vi "Pump waveplate.vi"(0 "VISA Refnum in":refnum<visa-resource-name>, 1 "Trigger rate \nat maximum":dbl, 2 "Mode":enum16{"Constant power", "Constant time"}(ring), 3 "Trigger rate warnings?":bool, 5 "Target trial \nlength (ms)":dbl, 7 "Target trigger rate":dbl, 8 "Threshold":dbl, 9 "Photon #":i32, 11 "error in (no error)":errorcluster, 12 "appended array":dbl[][](array[numeric]), 13 "N":i32=5, 14 "Axis in":i32=3) -> (4 "VISA Refnum out":refnum<visa-resource-name>, 6 "Current position (units)":dbl, 10 "WP Error":bool=TRUE, 15 "error out":errorcluster)   [LabVIEW 2013]
uses:
  <vilib>/imath/engines/lvmath2/RunTimeEngine/NodeEndStatement/NIMS_NodeEndStatement_Output.vi
  <instcachedir>/0/NIMS_NodeEndStatement_Output_53EC0D466D134D7ABD903AC30B43404B.lvgen/NIMS_NodeEndStatement_Output_53EC0D466D134D7ABD903AC30B43404B_010.vi
  <instcachedir>/0/NIMS_NodeEndStatement_Output_53EC0D466D134D7ABD903AC30B43404B.lvgen/NIMS_NodeEndStatement_Output_53EC0D466D134D7ABD903AC30B43404B_009.vi
  <vilib>/imath/engines/lvmath2/RunTimeEngine/BuiltInFunctions/asin/NIMS_asin(C).vi
  <instcachedir>/0/NIMS_asin(C)_73B68F6B04904A8785972686F67E90FD.lvgen/NIMS_asin(C)_73B68F6B04904A8785972686F67E90FD_001.vi
  <vilib>/imath/engines/lvmath2/RunTimeEngine/BuiltInFunctions/abs/NIMS_abs(signed).vi
  <instcachedir>/0/NIMS_abs(signed)_C4FCB8E6058B49B797C7C8D53CA5F6EC.lvgen/NIMS_abs(signed)_C4FCB8E6058B49B797C7C8D53CA5F6EC_002.vi
  <vilib>/imath/engines/lvmath2/RunTimeEngine/ErrorHandling/NIMS_Finalize Error.vi
  <instcachedir>/0/NIMS_NodeEndStatement_Output_53EC0D466D134D7ABD903AC30B43404B.lvgen/NIMS_NodeEndStatement_Output_53EC0D466D134D7ABD903AC30B43404B_001.vi
  <instcachedir>/0/NIMS_abs(signed)_C4FCB8E6058B49B797C7C8D53CA5F6EC.lvgen/NIMS_abs(signed)_C4FCB8E6058B49B797C7C8D53CA5F6EC_000.vi
panel:
  in  "Number of trials to skip":i32=10
  out "Calculated trial length":dbl
  out "angle":dbl
  out "theta1":dbl
  out "t_ratio":dbl
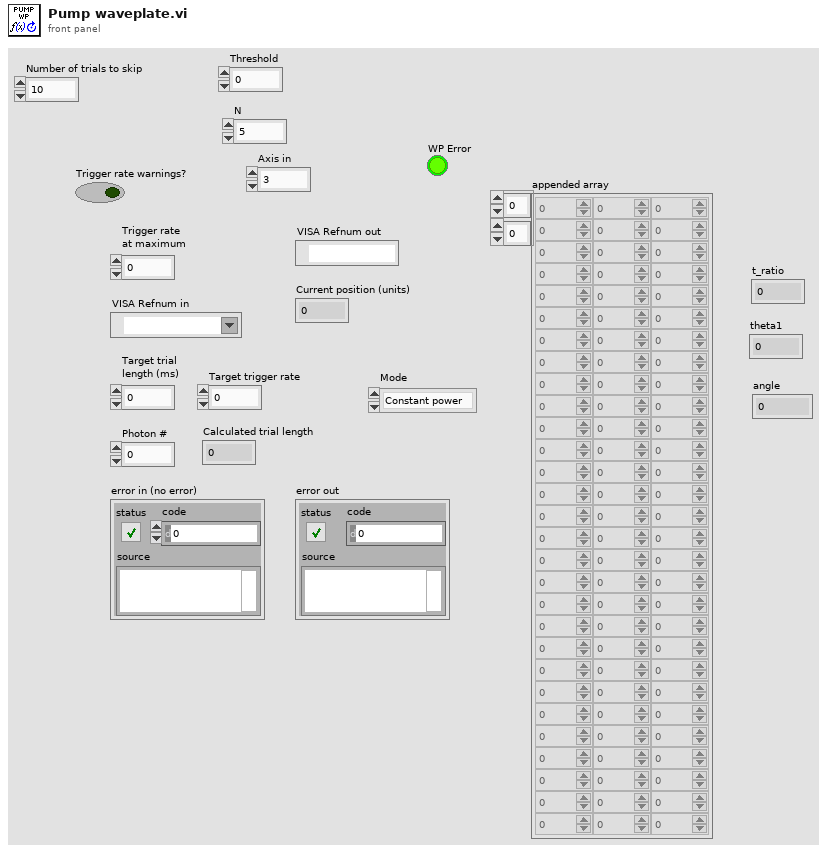
[diagram p1: front panel]
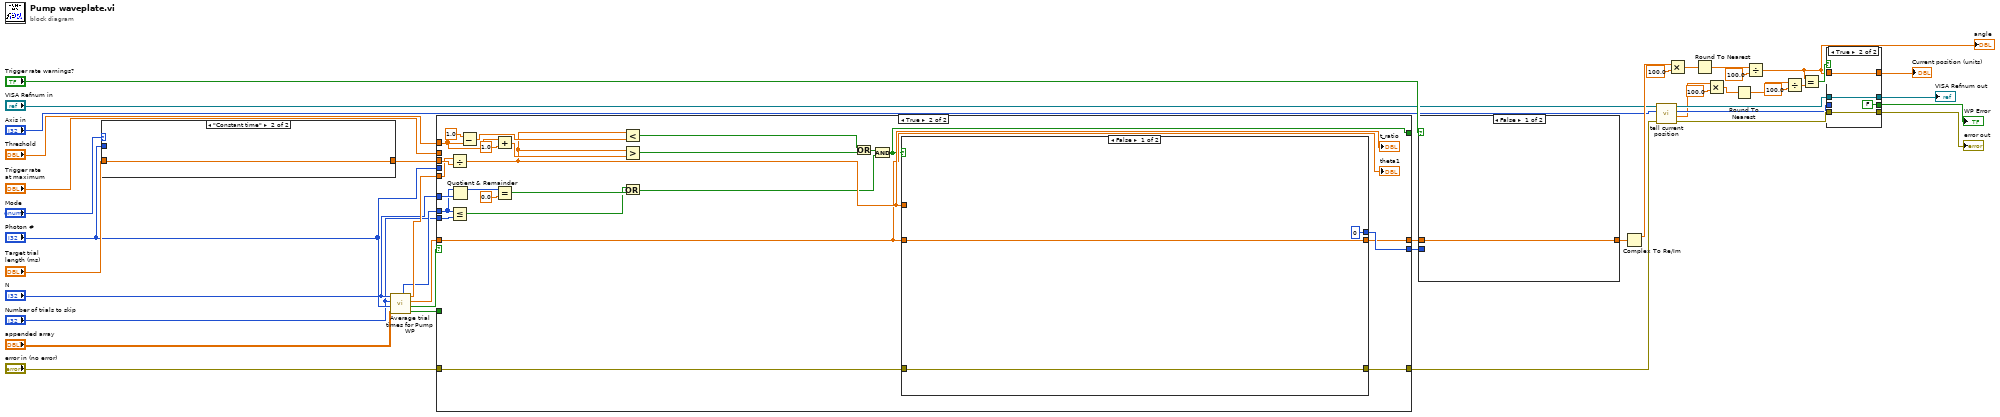
[diagram p0: block diagram]
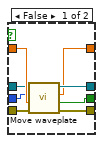
[diagram p2: hidden frame]
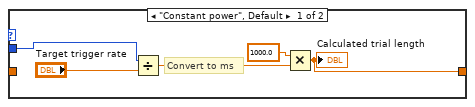
[diagram p3: hidden frame]
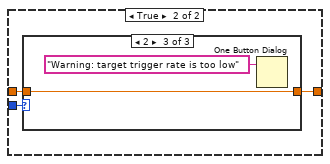
[diagram p4: hidden frame]
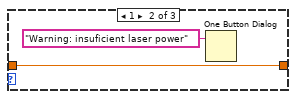
[diagram p6: hidden frame]
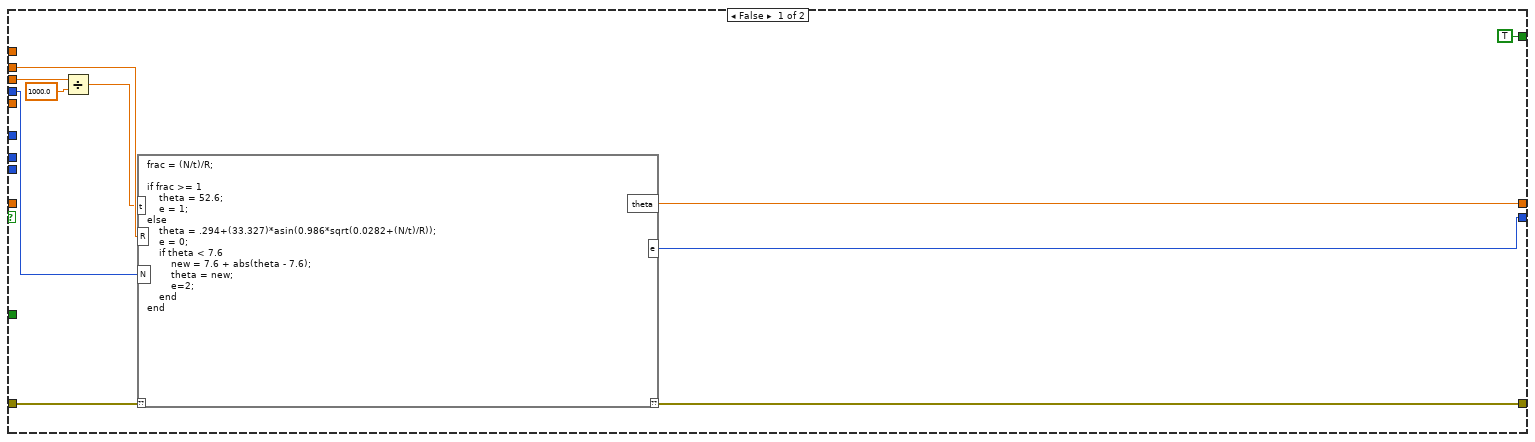
[diagram p7: hidden frame]
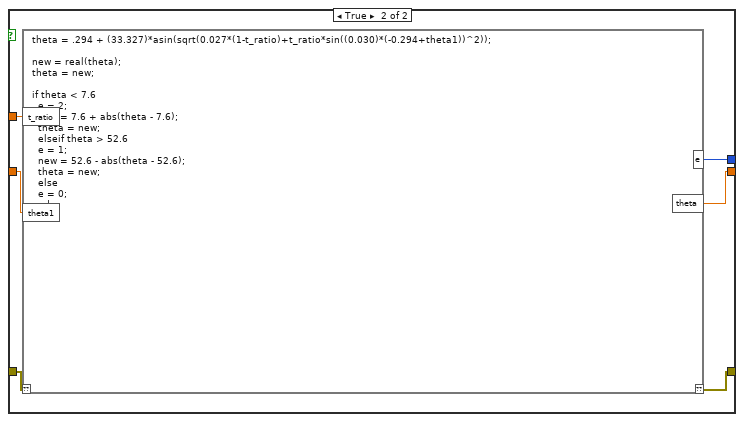
[diagram p8: hidden frame]
diagram:
  n1 = case shown="\"Constant time\"" "Mode" {
    tunnel: [w43 w48] -> w27
    tunnel: "Target trial \nlength (ms)" -> [_ w48]
    tunnel: "Photon #" -> [w47 _]
    frame "Constant power", Default {
      # "Convert to ms"
      n2 = Divide(x=w47, y="Target trigger rate") -> (x/y=w45:dbl)
      n3 = Multiply(x=1000.0, y=w45) -> (x*y=w43:dbl)
      "Calculated trial length" <- w43
    }
    frame "Constant time" {
    }
  }
  n4 = call "Average trial times for Pump WP.vi"("appended array"="appended array", "Photon #"="Photon #", "Number of trials to skip"="Number of trials to skip", "N"="N") -> ("At least N+1 values?"=w21:bool, "At least 1 value?"=w20:bool, "Last WP angle"=w19:dbl, "Output"=w18:dbl, "Number of values with specified photon #"=w17:i16)  [unwired: 1 in]
  n5 = case shown="True" w20 {
    tunnel: "Trigger rate \nat maximum" -> [w58 _]
    tunnel: [w50 w195] -> w39
    tunnel: [w57 w198] -> w41
    tunnel: w27 -> [w52 w199]
    tunnel: "Photon #" -> [w56 _]
    tunnel: "error in (no error)" -> [w55 w197]
    tunnel: [w54 w196] -> w14
    tunnel: "Threshold" -> [_ w191]
    tunnel: w21 -> [_ _]
    tunnel: w19 -> [_ w185]
    tunnel: w18 -> [_ w189]
    tunnel: [TRUE w184] -> _
    tunnel: w17 -> [_ w177]
    tunnel: "N" -> [_ w180]
    tunnel: "Number of trials to skip" -> [_ w176]
    frame False {
      n6 = Divide(x=w52, y=1000.0) -> (x/y=w51:dbl)
      n7 = mathscript code="frac = (N/t)/R;\n\nif frac >= 1\n    theta = 52.6;\n    e = 1;\nelse\n    theta = .294+(33.327)*asin(0.986*sqrt(0.0282+(N/t)/R));\n    e = 0;\n    if theta < 7.6\n        new = 7.6 + abs(theta - 7.6);\n        theta = new;\n        e=2;\n    end\nend"("??"=w55, "t"=w51, "R"=w58, "N"=w56) -> ("??"=w54:errorcluster, "e"=w57:i32, "theta"=w50:cdb)
    }
    frame True {
      n8 = Divide(x=w189, y=w199) -> (x/y=w188:dbl)
      "t_ratio" <- w188
      n9 = Less Or Equal?(x=w177, y=w176) -> (x <= y?=w175:bool)
      n10 = Quotient & Remainder(x=w177, y=w180) -> (x-y*floor(x/y)=w182:i32)  [unwired: 1 out]
      n11 = Subtract(x=1.0 ("y"), y=w191) -> (x-y=w190:dbl)
      n12 = Add(x=w191, y=1.0) -> (x+y=w193:dbl)
      n13 = Equal?(x=w182, y=0.0) -> (x = y?=w179:bool)
      n14 = Less?(x=w188, y=w190) -> (x < y?=w186:bool)
      n15 = Greater?(x=w188, y=w193) -> (0:w187:bool)
      n16 = Or(x=w175, y=w179) -> (x .or. y?=w178:bool)
      n17 = Or(x=w186, y=w187) -> (x .or. y?=w183:bool)
      n18 = And(x=w183, y=w178) -> (x .and. y?=w184:bool)
      n19 = case shown="False" w184 {
        tunnel: w188 -> [_ w208]
        tunnel: [0 ("e") w207] -> w198
        tunnel: w197 -> [w201 w206]
        tunnel: [w201 w205] -> w196
        tunnel: [w200 w204] -> w195
        tunnel: w185 -> [w200 w203]
        frame False {
        }
        frame True {
          n20 = mathscript code="theta = .294 + (33.327)*asin(sqrt(0.027*(1-t_ratio)+t_ratio*sin((0.030)*(-0.294+theta1))^2));\n\nnew = real(theta);\ntheta = new;\n\nif theta < 7.6\n  e = 2;\n  new = 7.6 + abs(theta - 7.6);\n  theta = new;\n  elseif theta > 52.6\n  e = 1;\n  new = 52.6 - abs(theta - 52.6);\n  theta = new;\n  else\n  e = 0;\nend"("??"=w206, "t_ratio"=w208, "theta1"=w203) -> ("??"=w205:errorcluster, "e"=w207:i32, "theta"=w204:dbl)
        }
      }
      "theta1" <- w185
    }
  }
  n21 = case shown="False" "Trigger rate warnings?" {
    tunnel: [w336 w339] -> w38
    tunnel: w39 -> [w336 w338]
    tunnel: w41 -> [_ w337]
    frame False {
    }
    frame True {
      n22 = case shown="2" w337 {
        tunnel: w338 -> [w340 w341 w343]
        tunnel: [w340 w341 w343] -> w339
        frame 0, Default {
        }
        frame 1 {
          n23 = One Button Dialog(message="Warning: insuficient laser power") -> ()  [unwired: 1 in, 1 out]
        }
        frame 2 {
          n24 = One Button Dialog(message="Warning: target trigger rate is too low") -> ()  [unwired: 1 in, 1 out]
        }
      }
    }
  }
  n25 = Complex To Re/Im(x + iy=w38) -> (x=w37:dbl)  [unwired: 1 out]
  n26 = call "tell current position.vi"("error in"=w14, "Axis in"="Axis in", "VISA Handle in"="VISA Refnum in") -> ("error out"=w13:errorcluster, "Current position (units)"=w2:dbl, "Axis out"=w10:i32, "VISA Handle out"=w9:refnum<visa-resource-name>)  [unwired: 2 in, 1 out]
  n27 = Multiply(x=w37, y=100.0) -> (x*y=w35:dbl)
  n28 = Round To Nearest(number=w35) -> (nearest integer value=w34:dbl)
  n29 = Multiply(x=w2, y=100.0) -> (x*y=w5:dbl)
  n30 = Round To Nearest(number=w5) -> (nearest integer value=w4:dbl)
  n31 = Divide(x=w34, y=100.0) -> (x/y=w7:dbl)
  "angle" <- w7
  n32 = Divide(x=w4, y=100.0) -> (x/y=w1:dbl)
  n33 = Equal?(x=w7, y=w1) -> (x = y?=w8:bool)
  n34 = case shown="True" w8 {
    tunnel: w13 -> [w352 w356]
    tunnel: w7 -> [w351 w353]
    tunnel: w10 -> [w350 _]
    tunnel: w9 -> [w349 w354]
    tunnel: [w348 w354] -> w31
    tunnel: [w347 FALSE ("WP Error")] -> w30
    tunnel: [w346 w353] -> w29
    tunnel: [w345 w356] -> w28
    frame False {
      n35 = call "Move waveplate.vi"("error in (no error)"=w352, "Angle"=w351, "Axis in"=w350, "VISA Refnum in"=w349) -> ("error out"=w345:errorcluster, "WP Error"=w347:bool, "Current position (units)"=w346:dbl, "VISA Refnum out"=w348:refnum<visa-resource-name>)  [unwired: 4 in]
    }
    frame True {
    }
  }
  "Current position (units)" <- w29
  "error out" <- w28
  "VISA Refnum out" <- w31
  "WP Error" <- w30
